vi "Cervical_overlay_thickROI.vi"(6 "Color":u32[](array[colorbox])=[65280], 7 "Group":string, 8 "error in (no error)":errorcluster, 9 "Thickness":i32, 10 "ROI":T2 {"Contours"."Type" items=["No Selection", "Point", "Line", "Rectangle", "Oval", "Polygon", "Freehand Region", "Annulus", "Unused2", "Unused3", "Broken Line", "Freehand Line", "Rotated Rectangle"]}, 11 "Image":T1) -> (0 "error out":errorcluster, 3 "Image Out":T1)   [LabVIEW 2021]
uses:
  <vilib>/vision/Image Controls.llb/IMAQ Image.ctl
  <vilib>/vision/NI_Vision_Development_Module.lvlib
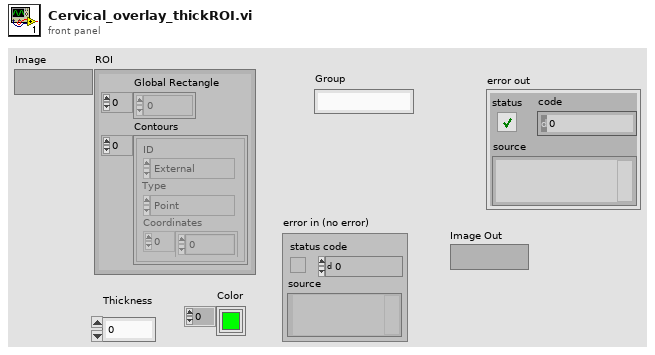
[diagram p1: front panel]
types:
  T1 = typedef "IMAQ Image.ctl" = refnum<image>
  T2 = typedef "ROI Descriptor" = cluster{"Global Rectangle":i32[], "Contours":cluster{"ID":enum32{"External", "Internal"}, "Type":u32, "Coordinates":i32[]}[]}
  T3 = enum32{"AutoM", "Close", "Dilate", "Erode", "Gradient", "Gradient in", "Gradient out", "HitMiss", "Open", "PClose", "POpen", "Thick", "Thin"}
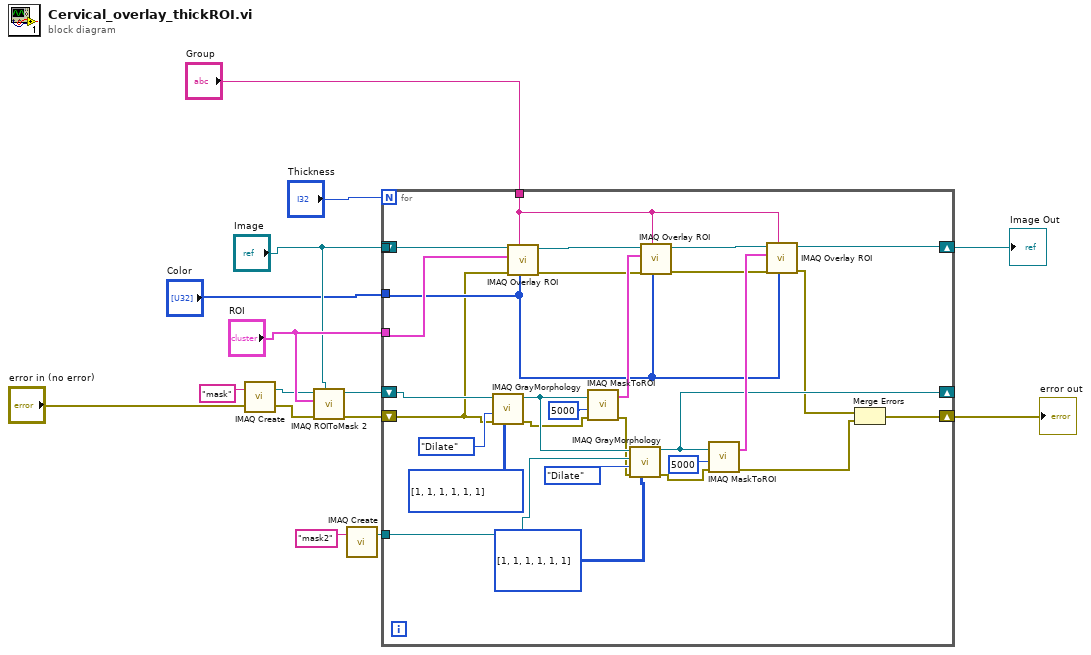
[diagram p0: block diagram]
diagram:
  n1 = call "IMAQ Create"("Image Name"="mask", "error in (no error)"="error in (no error)") -> ("New Image"=w11:T1, "error out"=w3:errorcluster)  [unwired: 3 in]
  n2 = call "IMAQ ROIToMask 2"("Image Model"="Image", "error in (no error)"=w3, "ROI Descriptor"="ROI", "Image"=w11) -> ("error out"=w2:errorcluster, "Image Out"=w10:T1)  [unwired: 5 in, 1 out]
  n3 = call "IMAQ Create"("Image Name"="mask2") -> ("New Image"=w8:T1)  [unwired: 4 in, 1 out]
  n4 = for {
    N: "Thickness" -> [_]
    tunnel: "Image" -> [w34]
    tunnel: "ROI" -> [w33]
    tunnel: "Color" -> [w32]
    shift-right: [w30] -> w14
    shift-left: _ -> [_]
    shift-right: [w26] -> _
    shift-left: w10 -> [w29]
    tunnel: w8 -> [w27]
    tunnel: "Group" -> [w25]
    shift-right: [w20] -> w1
    shift-left: w2 -> [w19]
    n5 = call "IMAQ GrayMorphology"("Structuring Element"=i32[][] [[1, 1, 1], [1, 1, 1]], "error in (no error)"=w19, "Operation"=T3."Dilate", "Image Src"=w29) -> ("error out"=w24:errorcluster, "Image Dst Out"=w28:T1)  [unwired: 6 in]
    n6 = call "IMAQ Overlay ROI"("Colors (Green)"=w32, "Group"=w25, "error in (no error)"=w19, "ROI Descriptor"=w33, "Image"=w34) -> ("error out"=w18:errorcluster, "Image Out"=w43:T1)  [unwired: 5 in]
    n7 = call "IMAQ MaskToROI"("Image"=w28, "Max number of vectors in ROI"=5000, "error in (no error)"=w24) -> ("ROI Descriptor"=w35:T2, "error out"=w23:errorcluster)  [unwired: 4 in, 1 out]
    n8 = call "IMAQ GrayMorphology"("Structuring Element"=i32[][] [[1, 1], [1, 1], [1, 1]], "error in (no error)"=w23, "Operation"=T3."Dilate", "Image Dst"=w27, "Image Src"=w28) -> ("error out"=w22:errorcluster, "Image Dst Out"=w26:T1)  [unwired: 5 in]
    n9 = call "IMAQ Overlay ROI"("Colors (Green)"=w32, "Group"=w25, "error in (no error)"=w18, "ROI Descriptor"=w35, "Image"=w43) -> ("error out"=w17:errorcluster, "Image Out"=w31:T1)  [unwired: 5 in]
    n10 = call "IMAQ MaskToROI"("Image"=w26, "Max number of vectors in ROI"=5000, "error in (no error)"=w22) -> ("ROI Descriptor"=w42:T2, "error out"=w21:errorcluster)  [unwired: 4 in, 1 out]
    n11 = call "IMAQ Overlay ROI"("Colors (Green)"=w32, "Group"=w25, "error in (no error)"=w17, "ROI Descriptor"=w42, "Image"=w31) -> ("error out"=w16:errorcluster, "Image Out"=w30:T1)  [unwired: 5 in]
    n12 = Merge Errors(w16, w21) -> (w20:errorcluster)
  }
  "Image Out" <- w14
  "error out" <- w1
